vi "CalculateModeArray.vi"(8 "General settings":T4, 11 "Holo Settings":T1) -> (2 "ModeArray":dbl[][](array[numeric]))   [LabVIEW 2018]
uses:
  Controls/General Setting.ctl
  Controls/Buttons/Running Button.ctl
  Controls/Holo Setting.ctl
  Controls/Zernike Polynominals.ctl
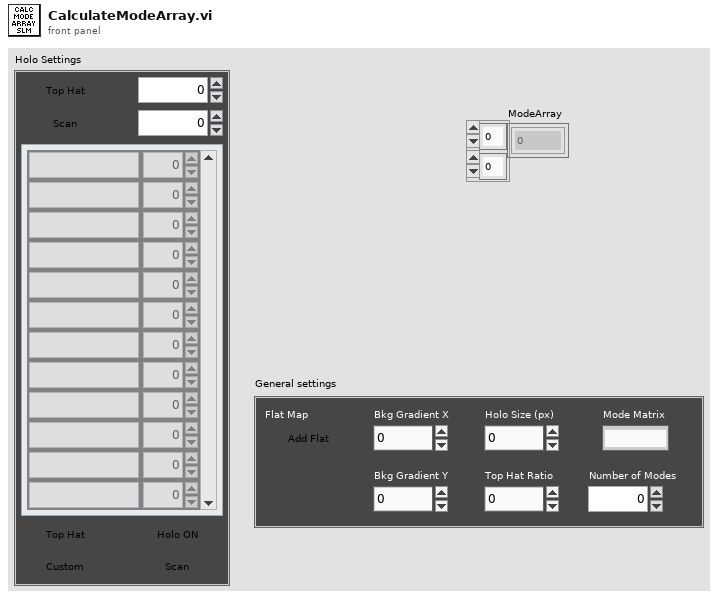
[diagram p1: front panel]
types:
  T1 = typedef "Holo Setting.ctl" = cluster{"Holo On":T2, "Scan":T2, "X":i16, "Y":i16, "Zernike Polynominals":T3, "Top Hat":T2, "Vortex":T2, "Clockwise":T2, "Custom":T2}
  T2 = typedef "Running Button.ctl" = bool
  T3 = typedef "Zernike Polynominals.ctl" = cluster{"Aberration Name":string, "Numeric":dbl}[]
  T4 = typedef "General Setting.ctl" = cluster{"Flat Map":T2, "Bkg Gradient X":dbl, "Bkg Gradient Y":dbl, "Holo Size (px)":i32, "Top Hat Ratio":dbl, "Number of Modes":i8, "Mode Matrix":u16}
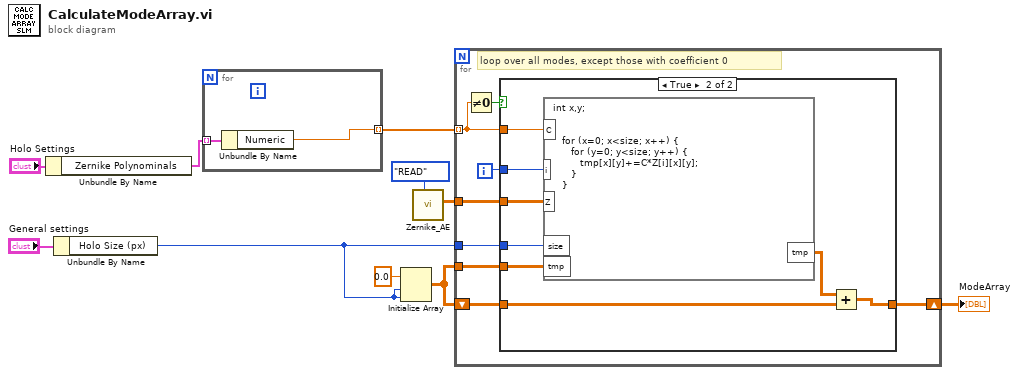
[diagram p0: block diagram]
diagram:
  n1 = Unbundle By Name("Holo Settings") -> ("Zernike Polynominals"=w3:T3)
  n2 = Unbundle By Name("General settings") -> ("Holo Size (px)"=w1:i32)
  n3 = for {
    tunnel: w3 -> [w12] mode=indexing
    tunnel: [w11] -> w2 mode=indexing
    n4 = Unbundle By Name(w12) -> ("Numeric"=w11:dbl)
  }
  n5 = Initialize Array(0.0 ("element"), w1, w1) -> (w8:dbl[][])
  n6 = call "Zernike_AE.vi"("Action"=enum16{"READ", "WRITE"}."READ") -> ("Zernike Out"=w6:dbl[][][])  [unwired: 10 in]
  n7 = for {
    shift-right: [w13] -> w10
    shift-left: w8 -> [w14]
    tunnel: w6 -> [w17]
    tunnel: w1 -> [w20]
    tunnel: w2 -> [w16] mode=indexing
    tunnel: w8 -> [w19]
    i -> [w18]
    # "loop over all modes, except those with coefficient 0"
    n8 = Not Equal To 0?(x=w16) -> (x != 0?=w15:bool)
    n9 = case shown="True" w15 {
      tunnel: w20 -> [_ w29]
      tunnel: w19 -> [_ w28]
      tunnel: w16 -> [_ w27]
      tunnel: w18 -> [_ w26]
      tunnel: w17 -> [_ w25]
      tunnel: w14 -> [w21 w23]
      tunnel: [w21 w22] -> w13
      frame False {
      }
      frame True {
        n10 = formula code="int x,y;\n\n\n   for (x=0; x<size; x++) {\n      for (y=0; y<size; y++) {\n         tmp[x][y]+=C*Z[i][x][y];\n      }\n   }"("C"=w27, "size"=w29, "tmp"=w28, "i"=w26, "Z"=w25) -> ("tmp"=w24:dbl[][])
        n11 = Add(x=w24, y=w23) -> (x+y=w22:dbl[][])
      }
    }
  }
  "ModeArray" <- w10
